vi "WRP Get Property Integer.vi"(8 "error in (no error)":errorcluster, 9 "size":i32, 10 "index":i32, 11 "property":string) -> (0 "error out":errorcluster, 1 "size out":i32, 2 "function return":i32, 3 "value":i32)   [LabVIEW 2018, in "SesWrapper.lvlib"]
doc: "int STDCALL WRP_GetPropertyInteger(const String property, int index, int *value, int *size);"
uses:
  SesWrapper.lvlib
  build/Debug/SESWrapper.dll
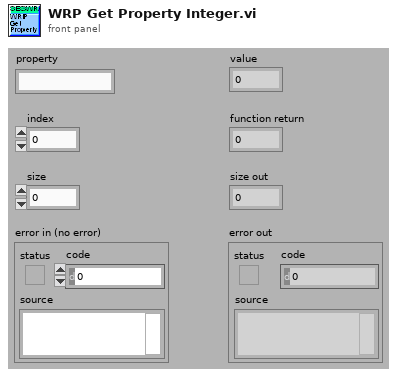
[diagram p1: front panel]
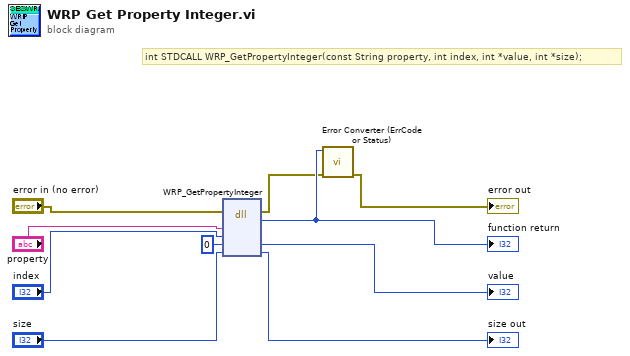
[diagram p0: block diagram]
diagram:
  # "int STDCALL WRP_GetPropertyInteger(const String property, int index, int *value, int *size);"
  n1 = dll-call lib="C:/Development/svn/seswrapper-lib/build/Debug/SESWrapper.*" fn="WRP_GetPropertyInteger"(error in="error in (no error)", "property"="property", "index"="index", "value"=0, "size"="size") -> (error out=w2:errorcluster, w10:i32, "value"=→"value":i32, "size"=→"size out":i32)  [unwired: 4 in, 1 out]
  "function return" <- w10
  n2 = call "Error Converter (ErrCode or Status).vi"("error in (no error)"=w2, "error code"=w10) -> ("error out"=→"error out":errorcluster)  [unwired: 9 in]
